vi "Set Report Font.vi"(0 "report in":refnum<class "NI_HTML.lvclass">, 1 "text color (unchanged)":u32(colorbox)=16777216, 2 "font settings source (VI Inputs)":u16(ring) items=["VI Inputs", "Font Dialog Box"], 5 "text options":T2, 9 "font settings":T3={"Charset (-1)"=-1, "Weight (-1)"=-1, "Name"="", "Size"=" "}, 11 "error in (no error)":errorcluster) -> (4 "report out":refnum<class "NI_HTML.lvclass">, 6 "font out":T1={"font name"="", "font size"=0.0, "bold"=0, "italic"=0, "underline"=0, "strike through"=0, "font color"=16777216} {"font size" format="%0.2f"; "strike through" items=["Unchanged", "Yes", "No"]; "underline" items=["Unchanged", "Yes", "No"]; "italic" items=["Unchanged", "Yes", "No"]; "bold" items=["Unchanged", "Yes", "No"]}, 15 "error out":errorcluster)   [LabVIEW 2015, in "NI_HTML.lvclass"]
doc: "Sets the font properties of the report, including those in the headers and footers."
uses:
  <vilib>/Utility/NIReport.llb/HTML/NI_HTML.lvclass
  <vilib>/Utility/NIReport.llb/font.ctl
  <vilib>/Utility/NIReport.llb/HTML/NI_HTML.lvclass/NI_HTML.ctl
  <vilib>/Utility/NIReport.llb/NI_ReportGenerationCore.lvlib
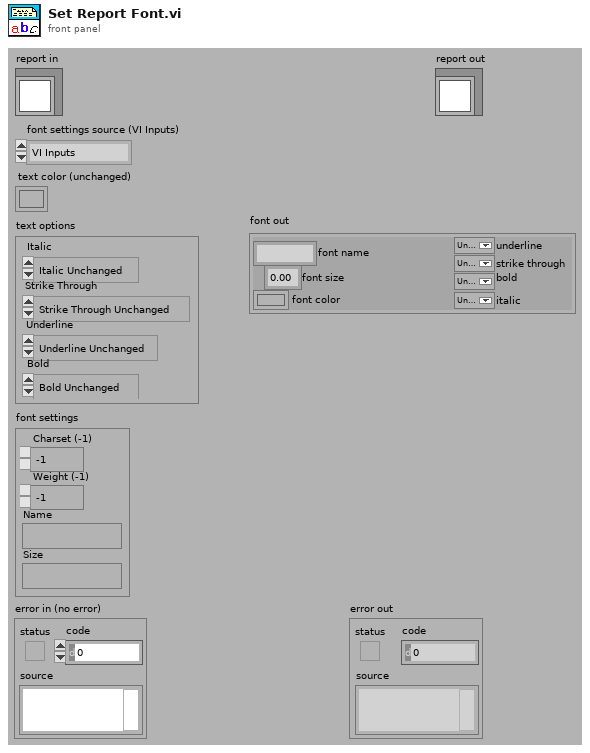
[diagram p1: front panel]
types:
  T1 = typedef "NI_ReportGenerationCore.lvlib/font.ctl" = cluster{"font name":string, "font size":dbl, "bold":u16, "italic":u16, "underline":u16, "strike through":u16, "font color":u32}
  T2 = cluster{"Italic":enum16{"Italic Unchanged", "Italic On", "Italic Off"}, "Strike Through":enum16{"Strike Through Unchanged", "Strike Through On", "Strike Through Off"}, "Underline":enum16{"Underline Unchanged", "Underline On", "Underline Off"}, "Bold":enum16{"Bold Unchanged", "Bold On", "Bold Off"}}
  T3 = cluster{"Charset (-1)":i16, "Weight (-1)":i16, "Name":string, "Size":string}
  T4 = typedef "NI_ReportGenerationCore.lvlib/HTML Report Data.ctl" = cluster{"Body Text":string, "Font Tag":string, "Title Text":string, "Header Text":string, "Footer Text":string, "Image List":path[]}
  T5 = typedef "NI_ReportGenerationCore.lvlib/Report Data Members.ctl" = cluster{"font":T1, "from template?":bool}
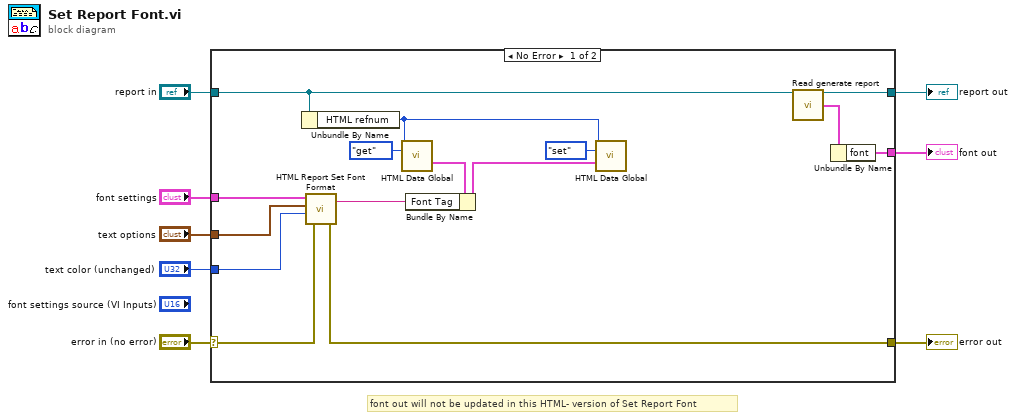
[diagram p0: block diagram]
diagram:
  # "font out will not be updated in this HTML- version of Set Report Font"
  n1 = case shown="No Error" "error in (no error)" {
    selector: "error in (no error)" -> [w19 w25]
    tunnel: [w18 w25] -> w7
    tunnel: [w16 w24] -> w5
    tunnel: "report in" -> [w13 w24]
    tunnel: "font settings" -> [w22 _]
    tunnel: "text options" -> [w21 _]
    tunnel: "text color (unchanged)" -> [w20 _]
    tunnel: [w17 _] -> w1
    frame No Error {
      n2 = Unbundle By Name(w13) -> ("HTML refnum"=w9:u32)
      n3 = call <vilib>:"HTML Report Set Font Format.vi"("Error In"=w19, "Text Color (unchanged)"=w20, "Text Options"=w21, "Font Settings"=w22) -> ("error out"=w18:errorcluster, "HTML formatting text"=w23:string)
      n4 = call <vilib>:"HTML Data Global.vi"("HTML refnum"=w9, "menu"=enum16{"init", "get", "set", "delete"}."get") -> ("HTML report data out"=w12:T4)  [unwired: 1 in, 12 out]
      n5 = Bundle By Name(cluster=w12, "Font Tag"=w23) -> (w10:T4)
      n6 = call <vilib>:"HTML Data Global.vi"("HTML refnum"=w9, "menu"=enum16{"init", "get", "set", "delete"}."set", "HTML report data in"=w10) -> ()  [unwired: 13 out]
      n7 = call-dynamic "Read generate report.vi"("report in"=w13) -> ("report out"=w16:refnum<class "NI_HTML.lvclass">, "generate report"=w15:T5)  [unwired: 1 in, 12 out]
      n8 = Unbundle By Name(w15) -> ("font"=w17:T1)
    }
    frame Error {
    }
  }
  "error out" <- w7
  "report out" <- w5
  "font out" <- w1
